vi "Vision Processing.vi"(4 "error in (no error)":errorcluster) -> ()   [LabVIEW 2015]
doc: "This VI runs in parallel to other tasks. It gets images from the camera, processes them for color or shape and use that information to affect robot behavior."
uses:
  <vilib>/Rock Robotics/WPI/Camera/WPI_CameraImageSize.ctl
  <vilib>/Rock Robotics/WPI/Camera/WPI_CameraWhite Balance Values.ctl
  <vilib>/Rock Robotics/WPI/Camera/WPI_CameraExposure Values.ctl
  <vilib>/Rock Robotics/WPI/Camera/WPI_CameraFrameRate.ctl
  Robot Global Data.vi
panel:
  in  "Drive Camera Image Size":T1=enum."320x240"
  # "VISION PROCESSING.VI"
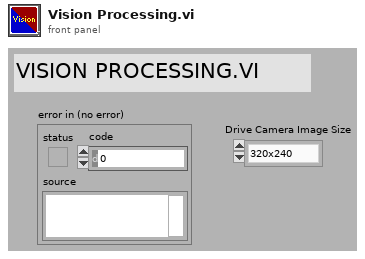
[diagram p1: front panel]
types:
  T1 = typedef "WPI_CameraImageSize.ctl" = enum16{"640x480", "320x240", "160x120", "Custom"}
  T2 = typedef "WPI_CameraFrameRate.ctl" = u32
  T3 = typedef "WPI_CameraExposure Values.ctl" = enum16{"Auto", "Flicker-free 50 Hz", "Flicker-free 60 Hz", "Hold current", "Custom"}
  T4 = typedef "WPI_CameraWhite Balance Values.ctl" = enum16{"Auto", "Fixed indoor", "Fixed outdoor 1", "Fixed outdoor 2", "Fixed fluorescent 1", "Fixed fluorescent 2", "Hold current", "Custom"}
  T5 = typedef "Image Type" = u32
  T6 = typedef "WPI_CameraDevRef.ctl" = cluster{"Camera Address":string, "CameraStatus":errorcluster}
  T7 = typedef "IMAQ Image.ctl" = refnum<image>
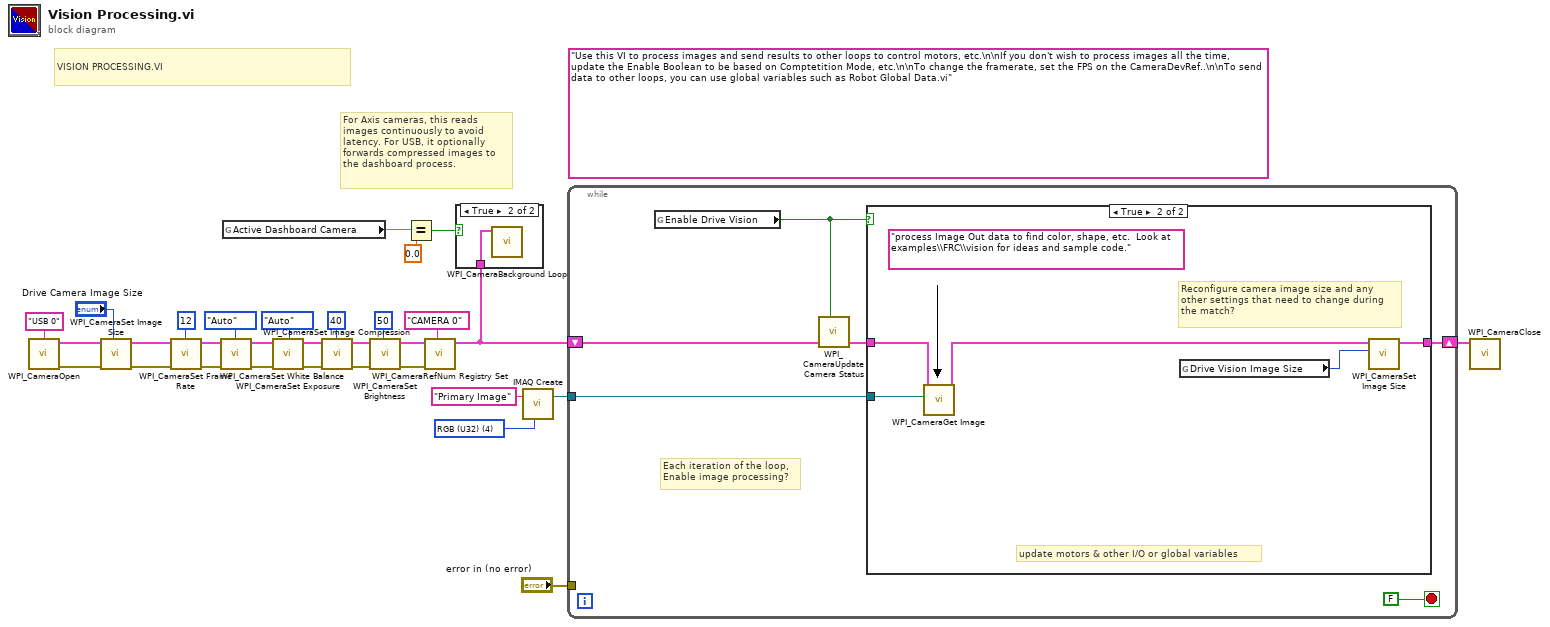
[diagram p0: block diagram]
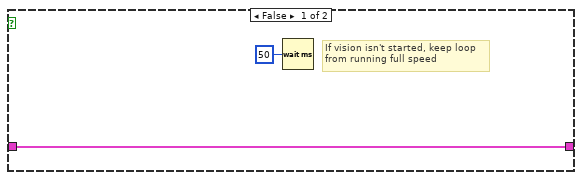
[diagram p3: hidden frame]
diagram:
  (unwired) "Use this VI to process images and send results to other loops to control motors, etc.\n\nIf you don't wish to process images all the time, update the Enable Boolean to be based on Comptetition Mode, etc.\n\nTo change the framerate, set the FPS on the CameraDevRef..\n\nTo send data to other loops, you can use global variables such as Robot Global Data.vi"
  w31 = T5 4 items=["Grayscale (U8)", "Grayscale (I16)", "Grayscale (SGL)", "Complex (CSG)", "RGB (U32)", "HSL (U32)", "RGB (U64)"] ("Image Type")
  # "VISION PROCESSING.VI"
  # "For Axis cameras, this reads\nimages continuously to avoid\nlatency. For USB, it optionally\nforwards compressed images to\nthe dashboard process."
  n1 = call <vilib>:"WPI_CameraOpen.vi"("Camera Address"="USB 0" ("format string")) -> ("error out"=w18:errorcluster, "CameraDevRef"=w19:T6)  [unwired: 1 in, 8 out]
  n2 = call <vilib>:"WPI_CameraSet Image Size.vi"("error in (no error)"=w18, "Image Size"="Drive Camera Image Size", "CameraDevRef"=w19) -> ("error out"=w17:errorcluster, "CameraDevRef Out"=w20:T6)  [unwired: 1 in, 6 out]
  n3 = call <vilib>:"WPI_CameraSet Frame Rate.vi"("error in (no error)"=w17, "Frame Rate (fps)"=T2 12, "CameraDevRef"=w20) -> ("error out"=w16:errorcluster, "CameraDevRef Out"=w22:T6)  [unwired: 7 out]
  n4 = call <vilib>:"WPI_CameraSet White Balance.vi"("error in (no error)"=w16, "White Balance"=WPI_CameraWhite_Balance_Values."Auto", "CameraDevRef"=w22) -> ("error out"=w15:errorcluster, "CameraDevRef Out"=w21:T6)  [unwired: 1 in, 6 out]
  n5 = global read "Robot Global Data.vi" "Active Dashboard Camera"() -> (w5:dbl)
  n6 = call <vilib>:"WPI_CameraSet Exposure.vi"("error in (no error)"=w15, "Exposure"=WPI_CameraExposure_Values."Auto", "CameraDevRef"=w21) -> ("error out"=w14:errorcluster, "CameraDevRef Out"=w24:T6)  [unwired: 1 in, 6 out]
  n7 = call <vilib>:"WPI_CameraSet Image Compression.vi"("error in (no error)"=w14, "Compression"=40, "CameraDevRef"=w24) -> ("error out"=w13:errorcluster, "CameraDevRef Out"=w23:T6)  [unwired: 7 out]
  n8 = call <vilib>:"WPI_CameraSet Brightness.vi"("error in (no error)"=w13, "Brightness"=50, "CameraDevRef"=w23) -> ("error out"=w11:errorcluster, "CameraDevRef Out"=w12:T6)  [unwired: 7 out]
  n9 = Equal?(x=w5, y=0.0) -> (x = y?=w3:bool)
  n10 = call <vilib>:"WPI_CameraRefNum Registry Set.vi"("error in (no error)"=w11, "refnum name"="CAMERA 0", "CameraDevRef"=w12) -> ("CameraDevRef"=w2:T6)  [unwired: 1 in, 7 out]
  n11 = case shown="True" w3 {
    tunnel: w2 -> [_ w32]
    frame False {
    }
    frame True {
      n12 = call <vilib>:"WPI_CameraBackground Loop.vi"("CameraDevRef"=w32) -> ()  [unwired: 11 in]
    }
  }
  n13 = call "IMAQ Create"("Image Name"="Primary Image", "Image Type"=w31) -> ("New Image"=w29:T7)  [unwired: 2 in, 2 out]
  n14 = while {
    shift-right: [w37] -> w28
    shift-left: w2 -> [w33]
    tunnel: w29 -> [w36]
    tunnel: "error in (no error)" -> [_]
    stop <- FALSE stop-if-true
    # "Each iteration of the loop,\nEnable image processing?"
    n15 = global read "Robot Global Data.vi" "Enable Drive Vision"() -> (w34:bool)
    n16 = call <vilib>:"WPI_CameraUpdate Camera Status.vi"("CameraDevRef In"=w33, "Enable Vision"=w34) -> ("CameraDevRef Out"=w35:T6)  [unwired: 3 in]
    n17 = case shown="True" w34 {
      tunnel: w36 -> [_ w44]
      tunnel: [w40 w45] -> w37
      tunnel: w35 -> [w40 w43]
      frame False {
        # "If vision isn't started, keep loop\nfrom running full speed"
        n18 = Wait (ms)(milliseconds to wait=u32 50) -> ()  [unwired: 1 out]
      }
      frame True {
        (unwired) "process Image Out data to find color, shape, etc.  Look at examples\\FRC\\vision for ideas and sample code."
        # "update motors & other I/O or global variables"
        # "Reconfigure camera image size and any\nother settings that need to change during\nthe match?"
        n19 = call <vilib>:"WPI_CameraGet Image.vi"("Image"=w44, "CameraDevRef"=w43) -> ("CameraDevRef Out"=w42:T6)  [unwired: 1 in, 8 out]
        n20 = global read "Robot Global Data.vi" "Drive Vision Image Size"() -> (w41:T1)
        n21 = call <vilib>:"WPI_CameraSet Image Size.vi"("Image Size"=w41, "CameraDevRef"=w42) -> ("CameraDevRef Out"=w45:T6)  [unwired: 2 in, 7 out]
      }
    }
  }
  n22 = call <vilib>:"WPI_CameraClose.vi"("CameraDevRef"=w28) -> ()  [unwired: 1 in, 10 out]
